vi "U3 Two 32-bit Frequency Measurements.vi"() -> ()   [LabVIEW 2021]
panel:
  in  "Case Constant\n(See Context Help)":bool=TRUE
  out "Frequency (FIO1)":dbl format="%.2f"
  out "Period (FIO1)":dbl format="%.6f"
  out "Iteration":i32
  out "Frequency (FIO0)":dbl format="%.2f"
  out "Period (FIO0)":dbl format="%.6f"
  in  "error in":errorcluster
  in  "Address":string="1"
  in  "FirstFound":bool=TRUE
  in  "stop":bool
  out "Counter1 Diff (FIO2)":u32
  out "error out":errorcluster
  out "Error Message":string
  # "Each iteration, this VI measures the frequency on FIO0 and FIO1 using timer mode 2 (32-bit\nperiod measurement).  Also reads the count on FIO2 and\ndisplays the difference from the previous iteration, with the idea that the same signal can\nbe connected to FIO0/FIO1 and FIO2 for comparison of period timing\nversus pulse counting."
  # "seconds"
  # "seconds"
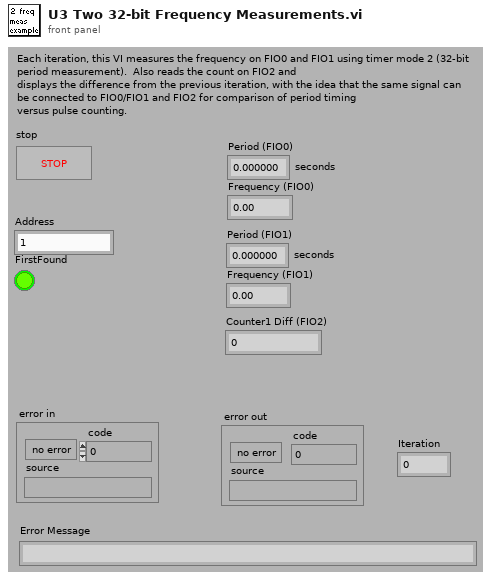
[diagram p1: front panel]
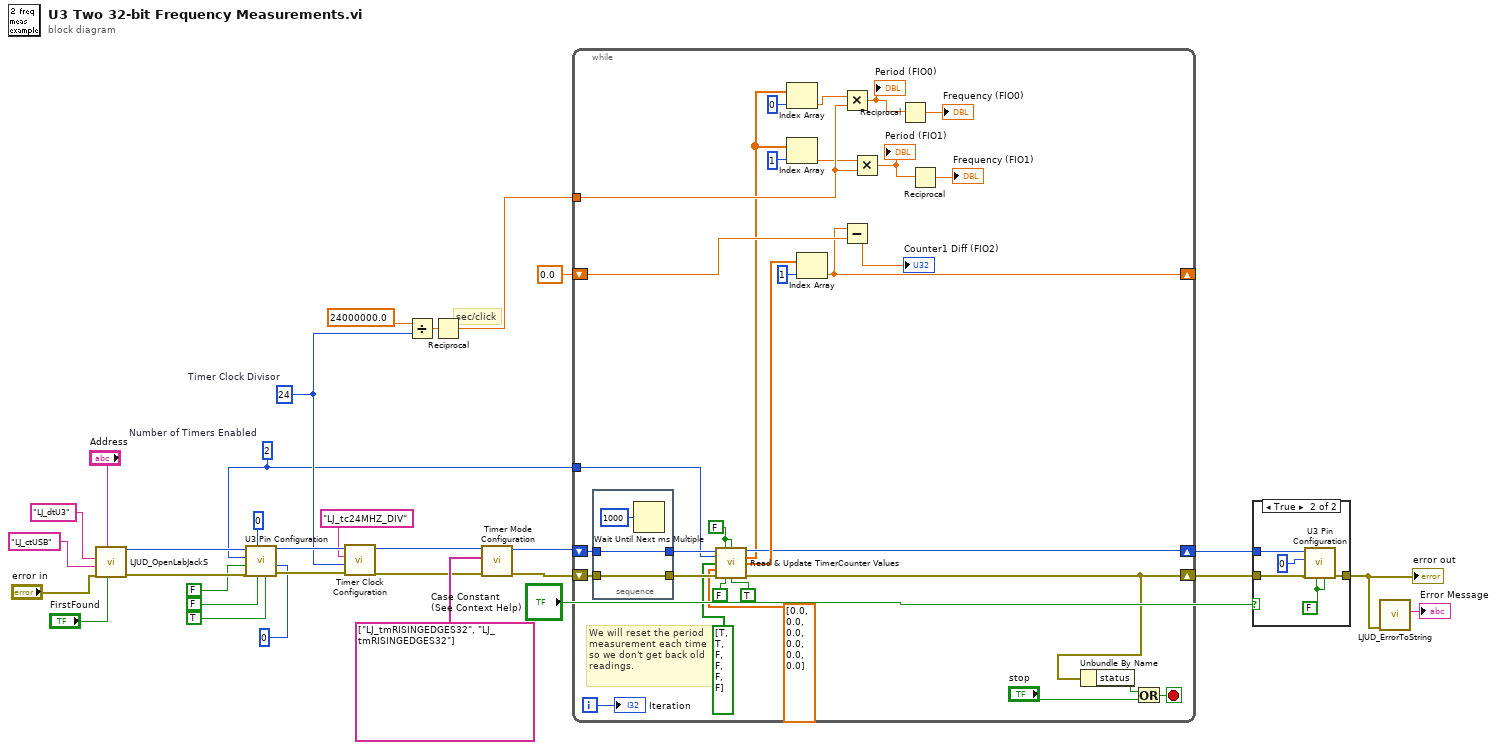
[diagram p0: block diagram]
diagram:
  w6 = 24  # Timer Clock Divisor
  w5 = u8 2  # Number of Timers Enabled
  # "sec/click"
  n1 = call "LJUD_OpenLabJackS.vi"("FirstFound"="FirstFound", "Address"="Address", "error in"="error in", "ConnectionType"="LJ_ctUSB", "DeviceType"="LJ_dtU3") -> ("error out"=w12:errorcluster, "Handle"=w13:i32)  [unwired: 4 in, 1 out]
  n2 = call "U3 Pin Configuration.vi"("Timer/Counter Pin Offset"=u8 0, "Enable Counter1"=TRUE ("Enable Counter0"), "Enable Counter0"=FALSE, "FIO/EIO Analog Enable"=0, "error in"=w12, "Enable DAC1"=FALSE ("Enable Counter0"), "Number of Timers Enabled"=w5, "Handle In"=w13) -> ("error out"=w16:errorcluster, "Handle Out"=w15:i32)  [unwired: 2 in]
  n3 = call "Timer Clock Configuration.vi"("error in"=w16, "Timer Clock Divisor"=w6, "Timer Clock Base"="LJ_tc24MHZ_DIV", "Handle In"=w15) -> ("error out"=w17:errorcluster, "Handle Out"=w14:i32)  [unwired: 6 in]
  n4 = Divide(x=24000000.0, y=w6) -> (x/y=w22:dbl)
  n5 = Reciprocal(x=w22) -> (1/x=w21:dbl)
  n6 = call "Timer Mode Configuration.vi"("error in"=w17, "TimerModes"=string[] ["LJ_tmRISINGEDGES32", "LJ_tmRISINGEDGES32"], "Handle In"=w14) -> ("error out"=w10:errorcluster, "Handle Out"=w11:i32)  [unwired: 7 in]
  n7 = while {
    shift-right: [w39] -> w27
    shift-left: w11 -> [w62]
    shift-right: [w38] -> w28
    shift-left: w10 -> [w61]
    tunnel: w21 -> [w42]
    shift-right: [w47] -> _
    shift-left: 0.0 ("TimerClockConfig") -> [w49]
    tunnel: w5 -> [w37]
    i -> [w46]
    stop <- w54 stop-if-true
    w60 = FALSE ("Reset Counter0")
    # "We will reset the period\nmeasurement each time\nso we don't get back old\nreadings."
    n8 = stacked-sequence {
      tunnel: [w64] -> w57
      tunnel: [w63] -> w56
      tunnel: w62 -> [w64]
      tunnel: w61 -> [w63]
      frame #0 {
        n9 = Wait Until Next ms Multiple(millisecond multiple=u32 1000) -> ()  [unwired: 1 out]
      }
    }
    n10 = call "Read & Update TimerCounter Values.vi"("Handle In"=w57, "Reset Counter0"=w60, "Reset Counter1"=w60, "# Timers to Read"=w37, "UpdateReset Timers"=bool[] [TRUE, TRUE, FALSE, FALSE, FALSE, FALSE], "TimerValues"=dbl[] [0.0, 0.0, 0.0, 0.0, 0.0, 0.0], "error in"=w56, "Read Counter0"=FALSE ("Reset Counter0"), "Read Counter1"=TRUE ("Reset Counter0")) -> ("Handle Out"=w39:i32, "Timer Value Reads"=w34:dbl[], "Counter Value Reads"=w59:dbl[], "error out"=w38:errorcluster)  [unwired: 3 in]
    n11 = Index Array(array=w34, index=0 ("Index")) -> (element=w43:dbl)
    n12 = Index Array(array=w34, index=1 ("Index")) -> (element=w36:dbl)
    n13 = Index Array(array=w59, index=1 ("Index")) -> (element=w47:dbl)
    n14 = Multiply(x=w43, y=w42) -> (x*y=w51:dbl)
    "Period (FIO0)" <- w51
    n15 = Subtract(x=w47, y=w49) -> (x-y=→"Counter1 Diff (FIO2)":dbl)
    n16 = Multiply(x=w36, y=w42) -> (x*y=w45:dbl)
    "Period (FIO1)" <- w45
    n17 = Reciprocal(x=w51) -> (1/x=→"Frequency (FIO0)":dbl)
    n18 = Reciprocal(x=w45) -> (1/x=→"Frequency (FIO1)":dbl)
    n19 = Unbundle By Name(w38) -> ("status"=w53:bool)
    n20 = Or(x=w53, y="stop") -> (x .or. y?=w54:bool)
    "Iteration" <- w46
  }
  n21 = case shown="True" "Case Constant\n(See Context Help)" {
    tunnel: w28 -> [w66 w71]
    tunnel: w27 -> [_ w70]
    tunnel: [w66 w67] -> w30
    frame False {
    }
    frame True {
      w69 = FALSE ("Enable Counter0")
      n22 = call "U3 Pin Configuration.vi"("Enable Counter1"=w69, "Enable Counter0"=w69, "error in"=w71, "Number of Timers Enabled"=u8 0 ("# Timers Enabled"), "Handle In"=w70) -> ("error out"=w67:errorcluster)  [unwired: 5 in, 1 out]
    }
  }
  "error out" <- w30
  n23 = call "LJUD_ErrorToString.vi"("error in"=w30) -> ("String"=→"Error Message":string)  [unwired: 10 in]
